vi "NF WF1973_74 FUNC User.vi"(6 "Read(F)":bool, 7 "Memory(1)":i32=1 min=0 max=128 step=1, 8 "error in (no error)":errorcluster caption="Error IN", 10 "Ch(Ch1)":bool, 11 "VISAsession":refnum<visa-resource-name>) -> (0 "error out":errorcluster caption="Error OUT", 2 "Query Memory":i32=999, 3 "CopyVISAsession":refnum<visa-resource-name>)   [LabVIEW 2010]
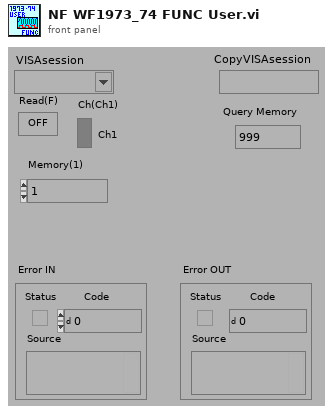
[diagram p1: front panel]
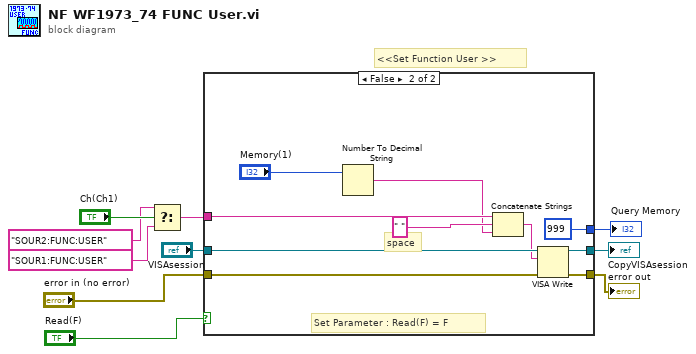
[diagram p0: block diagram]
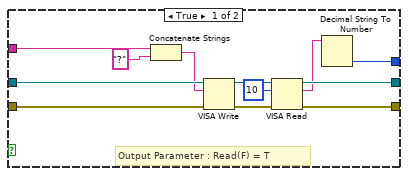
[diagram p2: hidden frame]
diagram:
  # "<<Set Function User >>"
  n1 = Select(t="SOUR2:FUNC:USER" ("文字列"), s="Ch(Ch1)", f="SOUR1:FUNC:USER" ("文字列")) -> (s? t:f=w3:string)
  n2 = case shown="FALSE" "Read(F)" {
    tunnel: "VISAsession" -> [w22 w32]
    tunnel: [w19 w30] -> w9
    tunnel: [w18 w31] -> w8
    tunnel: "error in (no error)" -> [w17 w26]
    tunnel: w3 -> [w15 w27]
    tunnel: [w11 999] -> w5
    frame True {
      # "Output Parameter : Read(F) = T"
      n3 = Concatenate Strings(w15, "?" ("形式文字列")) -> (w13:string)
      n4 = VISA Write(VISA resource name=w22, write buffer=w13, error in (no error)=w17) -> (VISA resource name out=w20:refnum<visa-resource-name>, error out=w21:errorcluster)  [unwired: 1 out]
      n5 = VISA Read(VISA resource name=w20, byte count=u32 10 ("バイトカウント（0）"), error in (no error)=w21) -> (VISA resource name out=w19:refnum<visa-resource-name>, read buffer=w12:string, error out=w18:errorcluster)  [unwired: 1 out]
      n6 = Decimal String To Number(string=w12) -> (number=w11:i32)  [unwired: 2 in, 1 out]
    }
    frame False {
      # "space"
      # "Set Parameter : Read(F) = F"
      n7 = Number To Decimal String(number="Memory(1)") -> (decimal integer string=w25:string)  [unwired: 1 in]
      n8 = Concatenate Strings(w27, " ", w25) -> (w29:string)
      n9 = VISA Write(VISA resource name=w32, write buffer=w29, error in (no error)=w26) -> (VISA resource name out=w30:refnum<visa-resource-name>, error out=w31:errorcluster)  [unwired: 1 out]
    }
  }
  "error out" <- w8
  "CopyVISAsession" <- w9
  "Query Memory" <- w5
